vi "Command Type.vi"(11 "Start Seq Command Config in":refnum<class "Start Seq Command Config.lvclass">) -> (2 "Command Type":T1)   [LabVIEW 2020, in "VolatusSeqConfig.lvlib" / "Start Seq Command Config.lvclass"]
uses:
  Start Seq Command Config.lvclass
  Start Seq Command Config.lvclass/Start Seq Command Config.ctl
  Command Type.ctl
  VolatusSeqConfig.lvlib
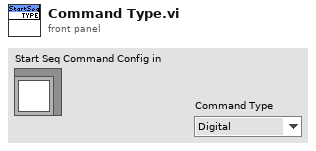
[diagram p1: front panel]
types:
  T1 = typedef "VolatusSeqConfig.lvlib/Command Type.ctl" = enum16{"Digital", "Numeric", "Transition", "Stop", "StartLog", "StopLog"}
  T2 = typedef "VolatusSeqConfig.lvlib/Command Type.ctl" = enum16{"Digital", "Numeric", "Transition", "Stop", "StartLog", "StopLog", "Start", "Event", "Error", "HTTP"}
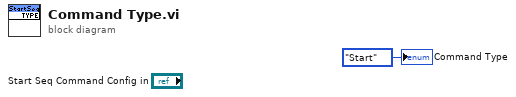
[diagram p0: block diagram]
diagram:
  "Command Type" <- Command_Type."Start" ("Command Type")
